vi "Read DAQmx device.vi"(8 "error in (no error)":errorcluster, 11 "DAQmx Base in":refnum<class "NI DAQmx Base.lvclass">) -> (0 "error out":errorcluster, 2 "DAQmx device":tag, 3 "DAQmx Base out":refnum<class "NI DAQmx Base.lvclass">)   [LabVIEW 2020, in "NI DAQmx.lvlib" / "NI DAQmx Base.lvclass"]
uses:
  NI DAQmx Base.lvclass
  NI DAQmx Base.lvclass/NI DAQmx Base.ctl
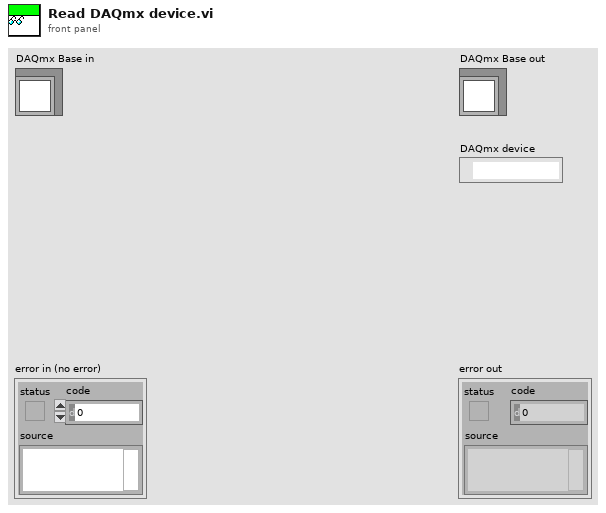
[diagram p1: front panel]
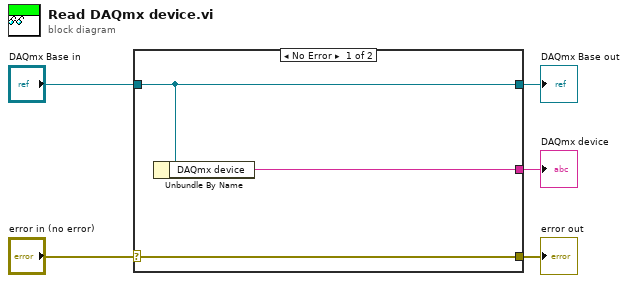
[diagram p0: block diagram]
diagram:
  n1 = case shown="No Error" "error in (no error)" {
    selector: "error in (no error)" -> [w8 w9]
    tunnel: [w8 w9] -> w4
    tunnel: [w7 w10] -> w2
    tunnel: "DAQmx Base in" -> [w7 w10]
    tunnel: [w6 _] -> w1
    frame No Error {
      n2 = Unbundle By Name(w7) -> ("DAQmx device"=w6:tag)
    }
    frame Error {
    }
  }
  "error out" <- w4
  "DAQmx Base out" <- w2
  "DAQmx device" <- w1
